vi "timeEstimate.vi"(6 "Cluster":T1, 9 "Exposure":dbl, 10 "Throwaway Frames":dbl, 11 "#Frames":dbl) -> (3 "Time":dbl)   [LabVIEW 2015]
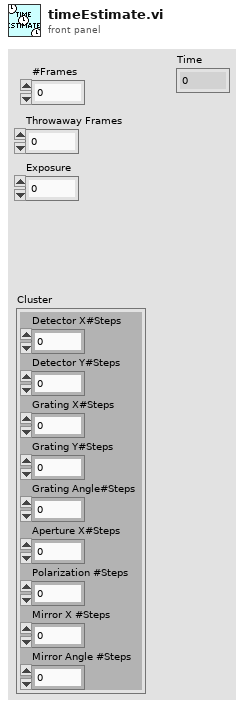
[diagram p1: front panel]
types:
  T1 = cluster{"Detector X#Steps":i32, "Detector Y#Steps":i32, "Grating X#Steps":i32, "Grating Y#Steps":i32, "Grating Angle#Steps":i32, "Aperture X#Steps":i32, "Polarization #Steps":i32, "Mirror X #Steps":i32, "Mirror Angle #Steps":i32}
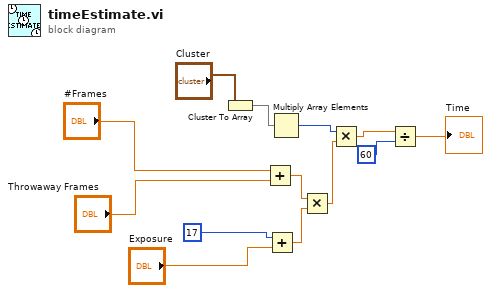
[diagram p0: block diagram]
diagram:
  n1 = Cluster To Array(cluster="Cluster") -> (array=w4:i32[])
  n2 = Add(x="#Frames", y="Throwaway Frames") -> (x+y=w7:dbl)
  n3 = Add(x=17, y="Exposure") -> (x+y=w8:dbl)
  n4 = Multiply Array Elements(1:w4) -> (0:w5:i32)
  n5 = Multiply(x=w7, y=w8) -> (x*y=w9:dbl)
  n6 = Multiply(x=w5, y=w9) -> (x*y=w10:dbl)
  n7 = Divide(x=w10, y=60) -> (x/y=→"Time":dbl)
